vi "send.vi"(7 "enqueue setting":T1, 8 "error in":errorcluster, 9 "timeout in ms (-1)":i32=-1, 10 "element":refnum<class "communicator message.lvclass">, 11 "communicator in":refnum<class "communicator.lvclass">) -> (0 "error out":errorcluster)   [LabVIEW 2015, in "communicator.lvclass"]
uses:
  communicator.lvclass
  message/communicator message.lvclass
  enqueue variety.ctl
  communicator.lvclass/communicator.ctl
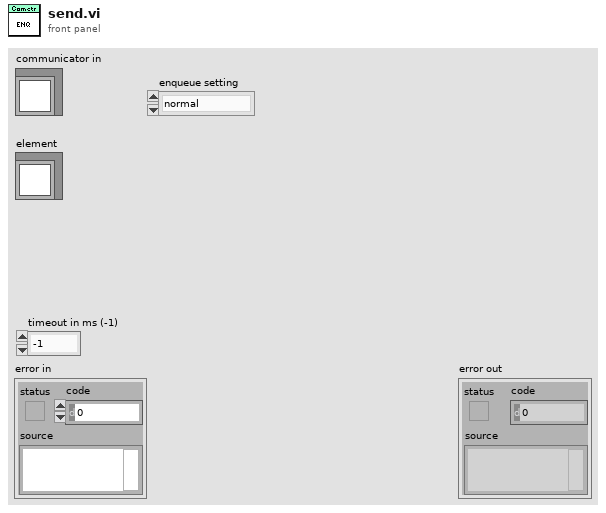
[diagram p1: front panel]
types:
  T1 = typedef "communicator.lvclass/enqueue variety.ctl" = enum16{"normal", "lossy", "priority"}
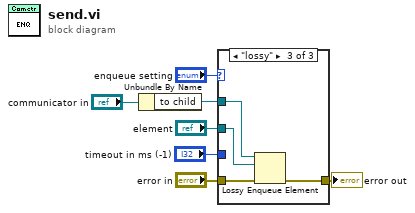
[diagram p0: block diagram]
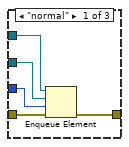
[diagram p2: hidden frame]
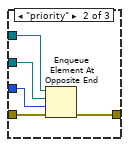
[diagram p3: hidden frame]
diagram:
  n1 = Unbundle By Name("communicator in") -> ("to child"=w6:refnum<queue>)
  n2 = case shown="\"lossy\"" "enqueue setting" {
    tunnel: w6 -> [w12 w17 w21]
    tunnel: "error in" -> [w11 w16 w18]
    tunnel: [w10 w15 w20] -> w4
    tunnel: "timeout in ms (-1)" -> [w9 w14 _]
    tunnel: "element" -> [w8 w13 w19]
    frame "normal" {
      n3 = Enqueue Element(queue=w12, element=w8, timeout in ms (-1)=w9, error in (no error)=w11) -> (error out=w10:errorcluster)  [unwired: 2 out]
    }
    frame "priority" {
      n4 = Enqueue Element At Opposite End(queue=w17, element=w13, timeout in ms (-1)=w14, error in (no error)=w16) -> (error out=w15:errorcluster)  [unwired: 2 out]
    }
    frame "lossy" {
      n5 = Lossy Enqueue Element(queue=w21, element=w19, error in (no error)=w18) -> (error out=w20:errorcluster)  [unwired: 3 out]
    }
  }
  "error out" <- w4
